vi "PPR_DRIVE_GET_SPEED_DEMAND.vi"() -> (1 "Right Wheel Limited Speed Dmd M/S":dbl format="%17.2f", 3 "Left Wheel Limited Speed Dmd M/S":dbl format="%17.2f")   [LabVIEW 2019]
uses:
  PPR_DRIVE_GLOBALS.vi
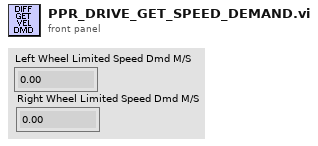
[diagram p1: front panel]
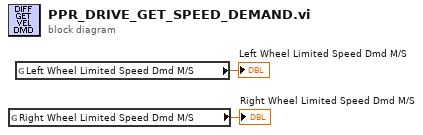
[diagram p0: block diagram]
diagram:
  n1 = global read "PPR_DRIVE_GLOBALS.vi" "Right Wheel Limited Speed Dmd M/S"() -> (→"Right Wheel Limited Speed Dmd M/S":dbl)
  n2 = global read "PPR_DRIVE_GLOBALS.vi" "Left Wheel Limited Speed Dmd M/S"() -> (→"Left Wheel Limited Speed Dmd M/S":dbl)
